vi "SetClassQueue.vi"(8 "ErrorIn(No Error)":errorcluster caption="entrée d'erreur (pas d'erreur)", 11 "OR77200.lvclass":refnum<class "OR77200.lvclass">) -> (0 "sortie d'erreur":errorcluster, 3 "OR77200.lvclass Out":refnum<class "OR77200.lvclass">)   [LabVIEW 2019, in "OR77200.lvclass"]
uses:
  OR77200.lvclass
  BaseDevice/BaseDevice.lvclass
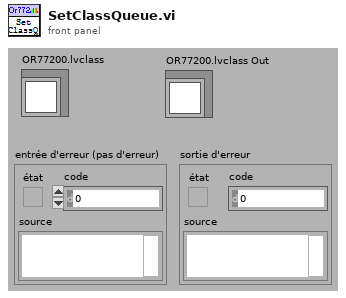
[diagram p1: front panel]
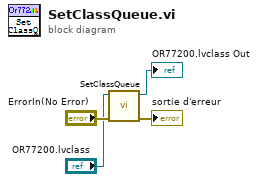
[diagram p0: block diagram]
diagram:
  n1 = call-parent "SetClassQueue.vi"("ErrorIn(No Error)"="ErrorIn(No Error)", "BaseDevice.lvclass"="OR77200.lvclass") -> ("sortie d'erreur"=→"sortie d'erreur":errorcluster, "BaseDevice.lvclass Out"=→"OR77200.lvclass Out":refnum<class "OR77200.lvclass">)  [unwired: 8 in]
